vi "Read Array.vi"(8 "error in (no error)":errorcluster, 11 "Doublo Array in":refnum<class "Doublo Array.lvclass">) -> (0 "error out":errorcluster, 2 "Array":dbl[](array[numeric]), 3 "Doublo Array out":refnum<class "Doublo Array.lvclass">)   [LabVIEW 2020, in "Example Source.lvlib" / "Doublo Array.lvclass"]
uses:
  Doublo Array.lvclass
  Doublo Array.lvclass/Doublo Array.ctl
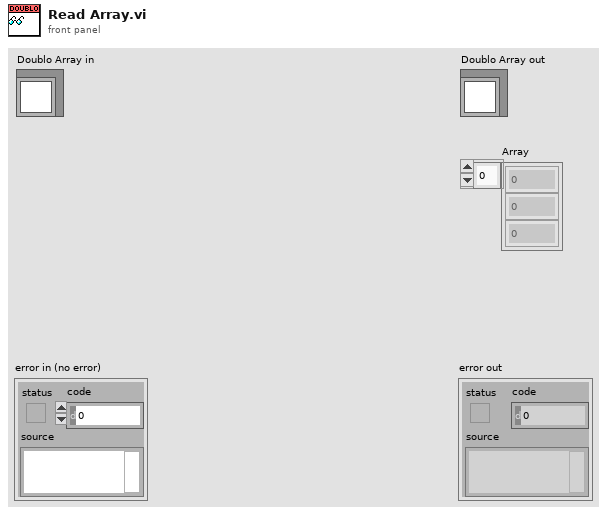
[diagram p1: front panel]
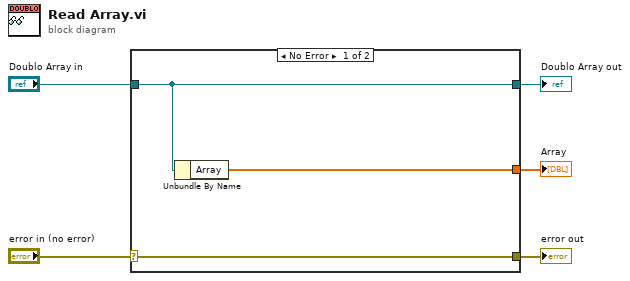
[diagram p0: block diagram]
diagram:
  n1 = case shown="No Error" "error in (no error)" {
    selector: "error in (no error)" -> [w8 w9]
    tunnel: [w8 w9] -> w4
    tunnel: [w7 w10] -> w2
    tunnel: "Doublo Array in" -> [w7 w10]
    tunnel: [w6 _] -> w1
    frame No Error {
      n2 = Unbundle By Name(w7) -> ("Array"=w6:dbl[])
    }
    frame Error {
    }
  }
  "error out" <- w4
  "Doublo Array out" <- w2
  "Array" <- w1
